vi "EXPT_CHEMOSTAT.vi"(4 "Load pump frequency":dbl, 7 "Loading program":T1(array[cluster]), 8 "error in (no error)":errorcluster, 10 "Buffer":dbl, 11 ".NET Refnum in":refnum<k24>) -> (0 "error out":errorcluster, 3 ".NET Refnum out":refnum<k24>)   [LabVIEW 2018]
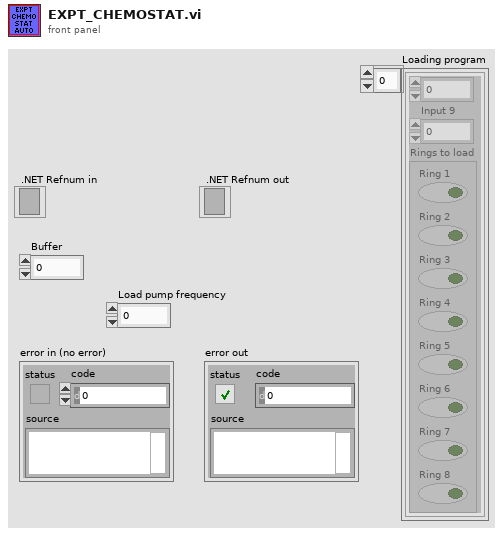
[diagram p1: front panel]
types:
  T1 = cluster{i32, "Input 9":dbl, "Rings to load":cluster{"Ring 1":bool, "Ring 2":bool, "Ring 3":bool, "Ring 4":bool, "Ring 5":bool, "Ring 6":bool, "Ring 7":bool, "Ring 8":bool}}[]
  T2 = cluster{"Ring 1":bool, "Ring 2":bool, "Ring 3":bool, "Ring 4":bool, "Ring 5":bool, "Ring 6":bool, "Ring 7":bool, "Ring 8":bool}
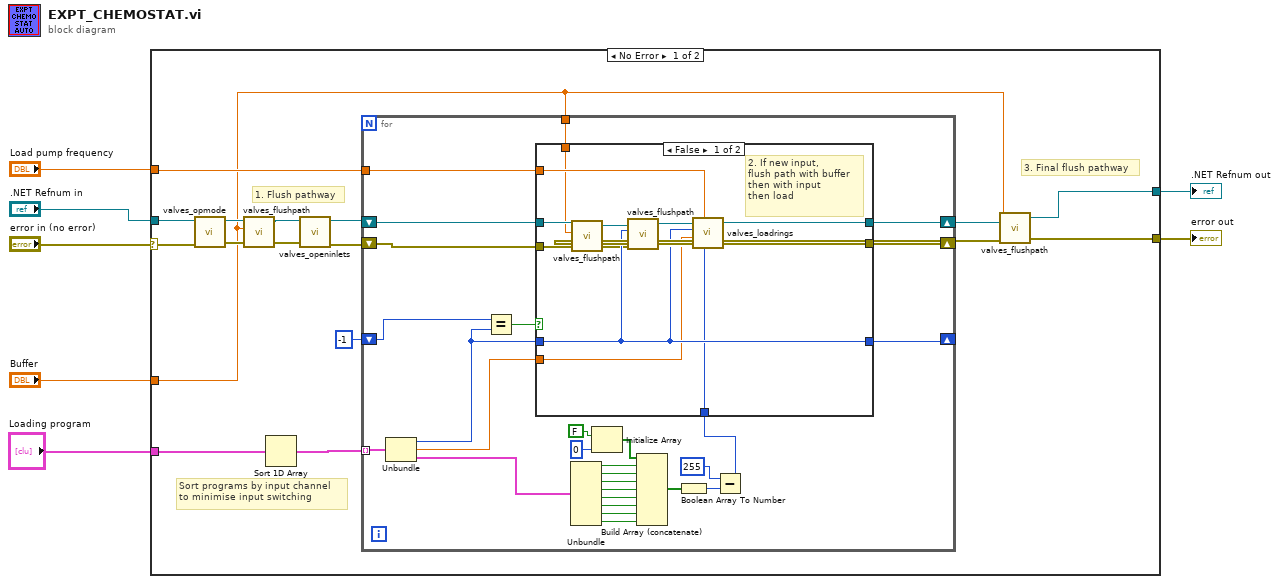
[diagram p0: block diagram]
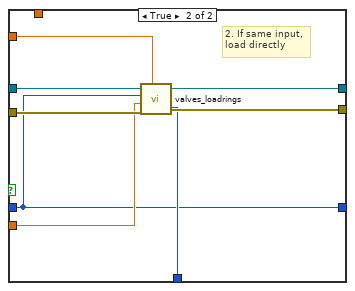
[diagram p2: hidden frame]
diagram:
  n1 = case shown="No Error" "error in (no error)" {
    selector: "error in (no error)" -> [w20 w74]
    tunnel: "Buffer" -> [w10 _]
    tunnel: [w19 w74] -> w5
    tunnel: ".NET Refnum in" -> [w18 w75]
    tunnel: [w17 w75] -> w7
    tunnel: "Load pump frequency" -> [w14 _]
    tunnel: "Loading program" -> [w13 _]
    frame No Error {
      # "3. Final flush pathway"
      # "1. Flush pathway"
      # "Sort programs by input channel\nto minimise input switching"
      n2 = call "valves_opmode.vi"("COM4 in"=w18, "error in"=w20) -> ("COM4 out"=w24:refnum<k24>, "error out"=w23:errorcluster)  [unwired: 5 in]
      n3 = call "valves_flushpath.vi"("COM4 in"=w24, "Input solution"=w10, "error in"=w23) -> ("COM4 out"=w9:refnum<k24>, "error out"=w8:errorcluster)  [unwired: 4 in]
      n4 = Sort 1D Array(array=w13) -> (sorted array=w12:T1)
      n5 = call "valves_openinlets.vi"("error in"=w8, "COM4 in"=w9) -> ("error out"=w15:errorcluster, "COM4 out"=w16:refnum<k24>)  [unwired: 4 in]
      n6 = for {
        tunnel: w14 -> [w48]
        shift-right: [w52] -> w22
        shift-left: w16 -> [w50]
        shift-right: [w51] -> w21
        shift-left: w15 -> [w49]
        tunnel: w12 -> [w47] mode=indexing
        shift-right: [w46] -> _
        shift-left: -1 -> [w44]
        tunnel: w10 -> [w25]
        n7 = Unbundle(w47) -> (w45:i32, "Input 9"=w42:dbl, "Rings to load"=w27:T2)
        n8 = Equal?(x=w44, y=w45) -> (x = y?=w43:bool)
        n9 = Unbundle(w27) -> ("Ring 1"=w41:bool, "Ring 2"=w40:bool, "Ring 3"=w39:bool, "Ring 4"=w38:bool, "Ring 5"=w37:bool, "Ring 6"=w36:bool, "Ring 7"=w35:bool, "Ring 8"=w34:bool)
        n10 = Initialize Array(FALSE, 0 ("dimension size")) -> (w28:bool[])
        n11 = Build Array (concatenate)(w28, w41, w40, w39, w38, w37, w36, w35, w34) -> (w29:bool[])
        n12 = Boolean Array To Number(Boolean array=w29) -> (number=w31:u32)
        n13 = Subtract(x=u32 255, y=w31) -> (x-y=w26:u32)
        n14 = case shown="False" w43 {
          tunnel: [w65 w70] -> w52
          tunnel: [w64 w72] -> w51
          tunnel: w50 -> [w55 w71]
          tunnel: w49 -> [w57 w73]
          tunnel: w48 -> [w61 w66]
          tunnel: [w60 w67] -> w46
          tunnel: w45 -> [w60 w67]
          tunnel: w42 -> [w59 w69]
          tunnel: w26 -> [w58 w68]
          tunnel: w25 -> [w53 _]
          frame False {
            # "2. If new input,\nflush path with buffer\nthen with input\nthen load"
            n15 = call "valves_flushpath.vi"("COM4 in"=w55, "Input solution"=w53, "error in"=w57) -> ("COM4 out"=w54:refnum<k24>, "error out"=w56:errorcluster)  [unwired: 4 in]
            n16 = call "valves_flushpath.vi"("COM4 in"=w54, "Input solution"=w60, "error in"=w56) -> ("COM4 out"=w63:refnum<k24>, "error out"=w62:errorcluster)  [unwired: 4 in]
            n17 = call "valves_loadrings.vi"("COM4 in"=w63, "Frequency"=w61, "Input solution"=w60, "Cycles"=w59, "Rings to open"=w58, "error in"=w62) -> ("COM4 out"=w65:refnum<k24>, "error out"=w64:errorcluster)  [unwired: 1 in]
          }
          frame True {
            # "2. If same input,\nload directly"
            n18 = call "valves_loadrings.vi"("COM4 in"=w71, "Frequency"=w66, "Input solution"=w67, "Cycles"=w69, "Rings to open"=w68, "error in"=w73) -> ("COM4 out"=w70:refnum<k24>, "error out"=w72:errorcluster)  [unwired: 1 in]
          }
        }
      }
      n19 = call "valves_flushpath.vi"("COM4 in"=w22, "Input solution"=w10, "error in"=w21) -> ("COM4 out"=w17:refnum<k24>, "error out"=w19:errorcluster)  [unwired: 4 in]
    }
    frame Error {
    }
  }
  "error out" <- w5
  ".NET Refnum out" <- w7
